vi "FTW-JSON-Construct-NewArray.vi"(11 "error in":errorcluster) -> (4 "JSON":refnum<class "FTW-Container.lvclass">, 15 "error out":errorcluster)   [LabVIEW 2015]
uses:
  container/FTW-Container.lvclass
panel:
  # "Inputs"
  # "Outputs"
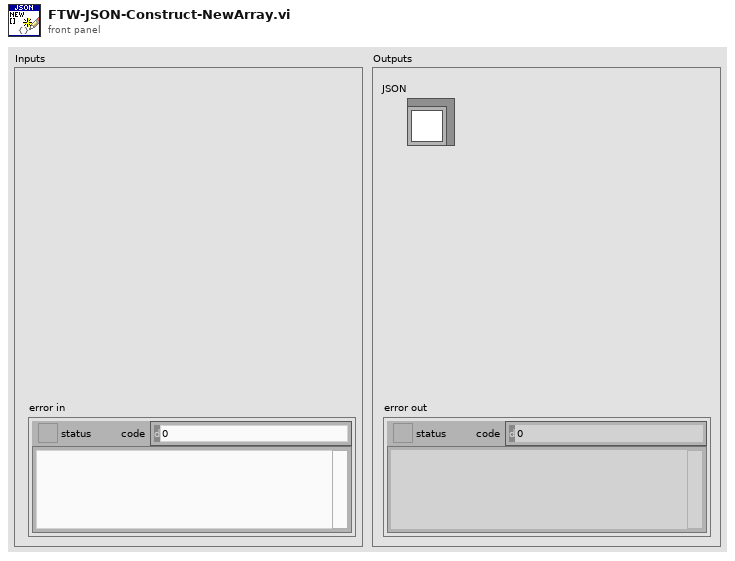
[diagram p1: front panel]
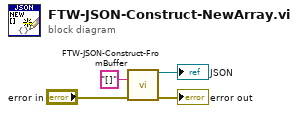
[diagram p0: block diagram]
diagram:
  n1 = call "FTW-JSON-Construct-FromBuffer.vi"("JSON String (UTF-8)"="[]", "error in"="error in") -> ("JSON"=→"JSON":refnum<class "FTW-Container.lvclass">, "error out"=→"error out":errorcluster)  [unwired: 12 in]
